vi "Raycaster_CalcInverseCameraMatrix.vi"(11 "Location Info":T1) -> (3 "Inverse Matrix":fxp<+/-,32,16>)   [LabVIEW 2020]
uses:
  Controls/Game_State.ctl
  Controls/Player_LocationInfo.ctl
  Controls/Player_LocationInfoAxis.ctl
  Controls/Map_Position.ctl
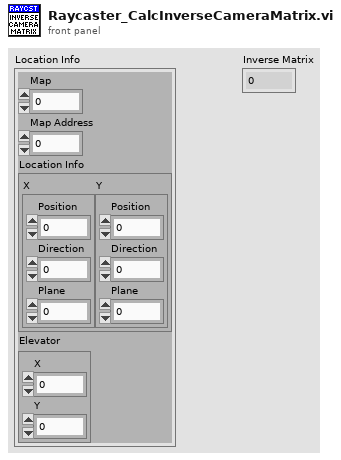
[diagram p1: front panel]
types:
  T1 = typedef "Game_State.ctl" = cluster{"Map":u8, "Map Address":u32, "Location Info":T2, "Elevator":T4}
  T2 = typedef "Player_LocationInfo.ctl" = cluster{"X":T3, "Y":T3}
  T3 = typedef "Player_LocationInfoAxis.ctl" = cluster{"Position":fxp<+/-,32,16>, "Direction":fxp<+/-,32,16>, "Plane":fxp<+/-,32,16>}
  T4 = typedef "Map_Position.ctl" = cluster{"X":fxp<+/-,32,16>, "Y":fxp<+/-,32,16>}
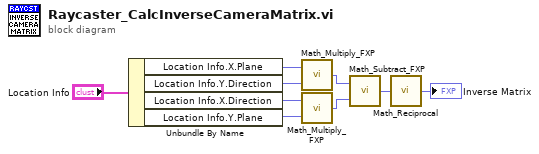
[diagram p0: block diagram]
diagram:
  n1 = Unbundle By Name("Location Info") -> ("Location Info.X.Plane"=w9:fxp<+/-,32,16>, "Location Info.Y.Direction"=w8:fxp<+/-,32,16>, "Location Info.X.Direction"=w6:fxp<+/-,32,16>, "Location Info.Y.Plane"=w7:fxp<+/-,32,16>)
  n2 = call "Math_Multiply_FXP.vi"("y"=w8, "x"=w9) -> ("x*y"=w5:fxp<+/-,32,16>)
  n3 = call "Math_Multiply_FXP.vi"("y"=w7, "x"=w6) -> ("x*y"=w4:fxp<+/-,32,16>)
  n4 = call "Math_Subtract_FXP.vi"("y"=w4, "x"=w5) -> ("x*y"=w3:fxp<+/-,32,16>)
  n5 = call "Math_Reciprocal.vi"("x"=w3) -> ("1/x"=→"Inverse Matrix":fxp<+/-,32,16>)
